vi "get_[]s2.vi"(7 "prefix":string, 11 "Array in":string[](array[string])) -> (3 "Array out":string[](array[string]))   [LabVIEW 2022 SP3]
uses:
  <vilib>/regexp/Match Regular Expression.xnode
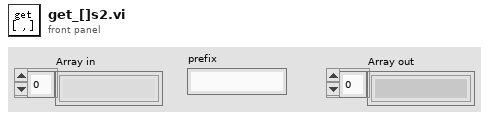
[diagram p1: front panel]
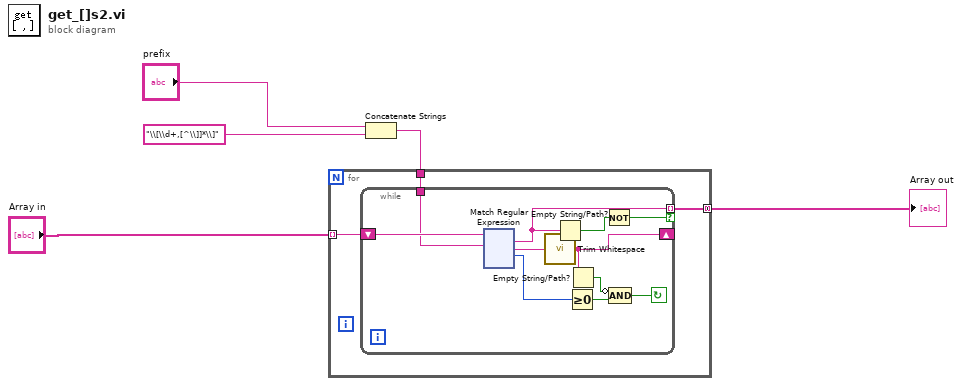
[diagram p0: block diagram]
diagram:
  n1 = Concatenate Strings("prefix", "\\[\\d+,[^\\]]*\\]" ("regular expression")) -> (w2:string)
  n2 = for {
    tunnel: "Array in" -> [w8] mode=indexing
    tunnel: [w7] -> w5 mode=concatenating
    tunnel: w2 -> [w6]
    n3 = while {
      shift-right: [w13] -> _
      shift-left: w8 -> [w16]
      tunnel: [w12] -> w7 mode=indexing if=w10
      tunnel: w6 -> [w9]
      stop <- w14 continue-if-true
      n4 = xnode "Match Regular Expression"("input string"=w16, "regular expression"=w9) -> ("whole match"=w12:string, "after match"=w18:string, "offset past match"=w15:i32)  [unwired: 4 in, 2 out]
      n5 = call <vilib>:"Trim Whitespace.vi"("string"=w18) -> ("trimmed string"=w13:string)  [unwired: 1 in]
      n6 = Empty String/Path?(string/path=w12) -> (empty?=w11:bool)
      n7 = Greater Or Equal To 0?(x=w15) -> (x >= 0?=w19:bool)
      n8 = Empty String/Path?(string/path=w13) -> (empty?=w17:bool)
      n9 = Not(x=w11) -> (.not. x?=w10:bool)
      n10 = Compound Arithmetic op=AND(invert w17, w19) -> (w14:bool)
    }
  }
  "Array out" <- w5
